vi "Tosca-Init Flags.vi"(0 "Tosca":refnum<class "Parameters.lvclass">) -> (4 "Tosca Out":refnum<class "Parameters.lvclass">, 8 "Names":string[](array[string]))   [LabVIEW 2020]
uses:
  Classes/Parameters/Parameters.lvclass
  Classes/Parameters/Parameters.lvclass/Parameters.ctl
  Classes/Parameters/Read Flags.vi
  Tosca-Globals.vi
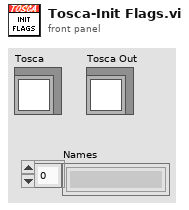
[diagram p1: front panel]
types:
  T1 = typedef "Tosca-Flag.ctl" = cluster{"Name":string, "Default":i32}
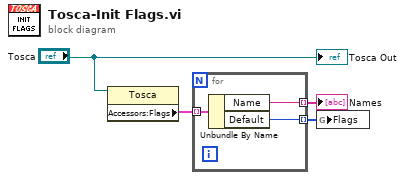
[diagram p0: block diagram]
diagram:
  n1 = property class="Tosca"(reference="Tosca") -> ("Accessors:Flags"=w1:T1[])  [unwired: 1 in, 2 out]
  n2 = for {
    tunnel: w1 -> [w7] mode=indexing
    tunnel: [w6] -> w4 mode=indexing
    tunnel: [w5] -> w3 mode=indexing
    n3 = Unbundle By Name(w7) -> ("Name"=w5:string, "Default"=w6:i32)
  }
  "Names" <- w3
  n4 = global write "Tosca-Globals.vi" "Flags"(w4) -> ()
  "Tosca Out" <- "Tosca"
